vi "Async Call Spawn Actor.vi"(7 "Actor":refnum<class "Actor.lvclass">, 10 "Spawn":refnum<class "Spawn.lvclass">) -> (0 "Error out":errorcluster)   [LabVIEW 2025, in "jettl.lvlib" / "Core Actor.lvlib" / "Core Actor.lvclass"]
uses:
  Core Actor.lvclass
  Actor/Actor.lvclass
  Spawn/Spawn/Spawn.lvclass
  Spawn Actor.vi
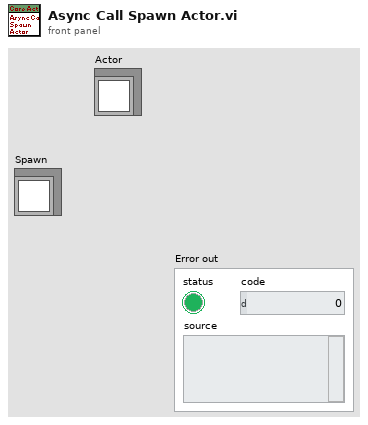
[diagram p1: front panel]
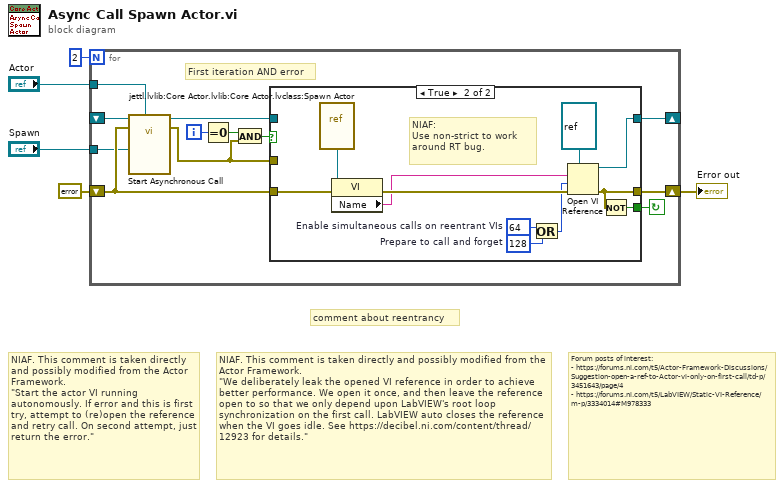
[diagram p0: block diagram]
diagram:
  # "Forum posts of interest:\n- https://forums.ni.com/t5/Actor-Framework-Discussions/Suggestion-open-a-ref-to-Actor-vi-only-on-first-call/td-p/3451643/page/4\n- https://forums.ni.com/t5/LabVIEW/Static-VI-Reference/m-p/3334014#M978333"
  # "NIAF. This comment is taken directly and possibly modified from the Actor Framework.\n\"We deliberately leak the opened VI reference in order to achieve better performance. We open it once, and then leave the reference open to so that we only depend upon LabVIEW's root loop synchronization on the first call. LabVIEW auto closes the reference when the VI goes idle. See https://decibel.ni.com/content/thread/12923 for details.\""
  # "NIAF. This comment is taken directly and possibly modified from the Actor Framework.\n\"Start the actor VI running autonomously. If error and this is first try, attempt to (re)open the reference and retry call. On second attempt, just return the error.\""
  # "comment about reentrancy"
  n1 = for {
    N: 2 -> [_]
    shift-right: [w17] -> _
    shift-left: _ -> [w16]
    shift-right: [w14] -> w2
    shift-left: errorcluster {"status"=FALSE, "code"=0, "source"=""} ("error out") -> [w10]
    tunnel: "Actor" -> [w7]
    tunnel: "Spawn" -> [w6]
    i -> [w12]
    stop <- w11 continue-if-true
    # "First iteration AND error"
    n2 = call-by-ref "Start Asynchronous Call"(reference=w16, error in=w10, "Actor in"=w7, "Spawn"=w6) -> (reference out=w15:refnum<vi>, error out=w8:errorcluster)  [unwired: 8 in, 2 out]
    n3 = Equal To 0?(x=w12) -> (x = 0?=w9:bool)
    n4 = And(x=w9, y=w8) -> (x .and. y?=w13:bool)
    n5 = case shown="True" w13 {
      tunnel: [w19 w28] -> w17
      tunnel: [w18 w26] -> w14
      tunnel: w15 -> [w19 _]
      tunnel: w8 -> [w18 _]
      tunnel: [_ w27] -> w11
      tunnel: w10 -> [_ w25]
      frame False {
      }
      frame True {
        w20 = 64  # Enable simultaneous calls on reentrant VIs
        w22 = 128  # Prepare to call and forget
        # "NIAF:\nUse non-strict to work around RT bug."
        n6 = vi-ref "jettl.lvlib:Core Actor.lvlib:Core Actor.lvclass:Spawn Actor.vi"() -> (w24:refnum<vi>)
        n7 = property class="VI"(reference=w24, error in=w25) -> (error out=w30:errorcluster, "Name"=w29:string)  [unwired: 1 out]
        n8 = Or(x=w20, y=w22) -> (x .or. y?=w21:i32)
        n9 = Open VI Reference(type specifier VI Refnum (for type only)=refnum<vi> refnum, vi path=w29, options=w21, error in (no error)=w30) -> (vi reference=w28:refnum<vi>, error out=w26:errorcluster)  [unwired: 2 in]
        n10 = Not(x=w26) -> (.not. x?=w27:bool)
      }
    }
  }
  "Error out" <- w2
